vi "Get Callers of Icon Editor Source Files.vi"() -> (0 "CallersOfIconEditorSourceFiles":path[](array[path]))   [LabVIEW 2020]
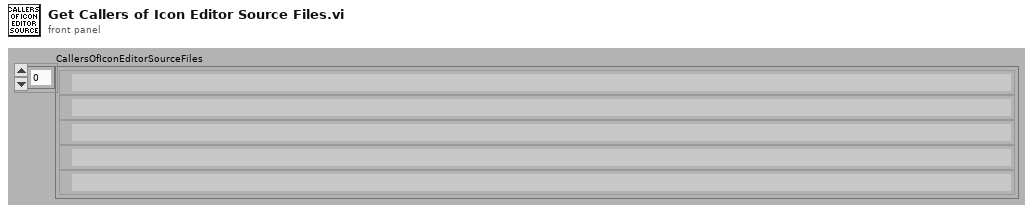
[diagram p1: front panel]
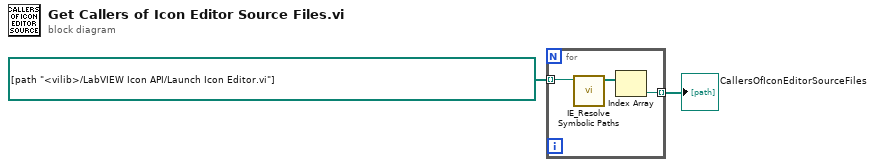
[diagram p0: block diagram]
diagram:
  n1 = for {
    tunnel: [w4] -> w2 mode=indexing
    tunnel: path[] [path "<vilib>/LabVIEW Icon API/Launch Icon Editor.vi"] ("Array") -> [w3] mode=indexing
    n2 = call "IE_Resolve Symbolic Paths.vi"("symbolic path"=w3) -> ("resolved paths"=w5:path[])  [unwired: 10 in]
    n3 = Index Array(array=w5) -> (element=w4:path)  [unwired: 1 in]
  }
  "CallersOfIconEditorSourceFiles" <- w2
